vi "control_potencia_lentes.vi"() -> ()   [LabVIEW 2024]
uses:
  TG JD - running/TG Juan Diego/Documentos de Labview/160620 Optotune Lens Driver 4 Labview package/Hello Optotune Lens (30.06.2015)/Calibration.ctl
  <vilib>/Instr/_visa.llb/VISA Configure Serial Port (Instr).vi
  <vilib>/Utility/file.llb/Write Delimited Spreadsheet (string).vi
panel:
  out "potencia  DER 3":dbl[](graph)
  in  "Número Usuario 2":string
  out "potencia  DER 2":dbl[](graph)
  out "potencia  DER":dbl[](graph)
  out "x+1":i32
  in  "stop":bool
  in  "Tab Control":enum32{"Experimento", "Configuración"}(tab)
  out "Grabando DATOS":bool
  out "path":path
  in  "Genero":string(combo)
  in  "Potencia inicial lente derecho":dbl(slide) scale=-3.0..3.0
  in  "Potencia inicial lente izquierdo":dbl(slide) scale=-3.0..3.0
  in  "VISA resource name 2":string="COM10"
  in  "VISA resource name":string="COM11"
  in  "Carpeta":path=path "C:/Users/TGM1603/Documents/LabVIEW Data/Experimentos electrodos"
  in  "Edad":string
  in  "Número Usuario":string
  in  "Hipermetropía (?)":string(combo)
  in  "Miopía (?)":string(combo)
  out "error out 4":errorcluster
  out "error out 3":errorcluster
  out "DPT  DER":dbl
  in  "stop 4":bool
  in  "error in (no error) 3":errorcluster
  in  "error in (no error) 4":errorcluster
  out "DPT  IZQ":dbl
  in  "stop 3":bool
  out "VISA resource name out 2":string
  out "Command to Port":string
  out "Data":string
  out "OK":bool
  out "Calibration 2":T1 {"Max Current A" format="%#_g mA"; "Max Current B" format="%#_g mA"; "UCL A" format="%#_g mA"; "LCL A" format="%#_g mA"; "UCL B" format="%#_g mA"; "LCL B" format="%#_g mA"}
  out "VISA resource name out":string
  out "ID":u16
  in  "Calibration":T1={"Max Current A"=293.0, "Max Current B"=293.0, "UCL A"=300.0, "UCL B"=300.0, "LCL A"=0.0, "LCL B"=0.0} {"Max Current A" format="%#_g mA"; "Max Current B" format="%#_g mA"; "UCL A" format="%#_g mA"; "LCL A" format="%#_g mA"; "UCL B" format="%#_g mA"; "LCL B" format="%#_g mA"}
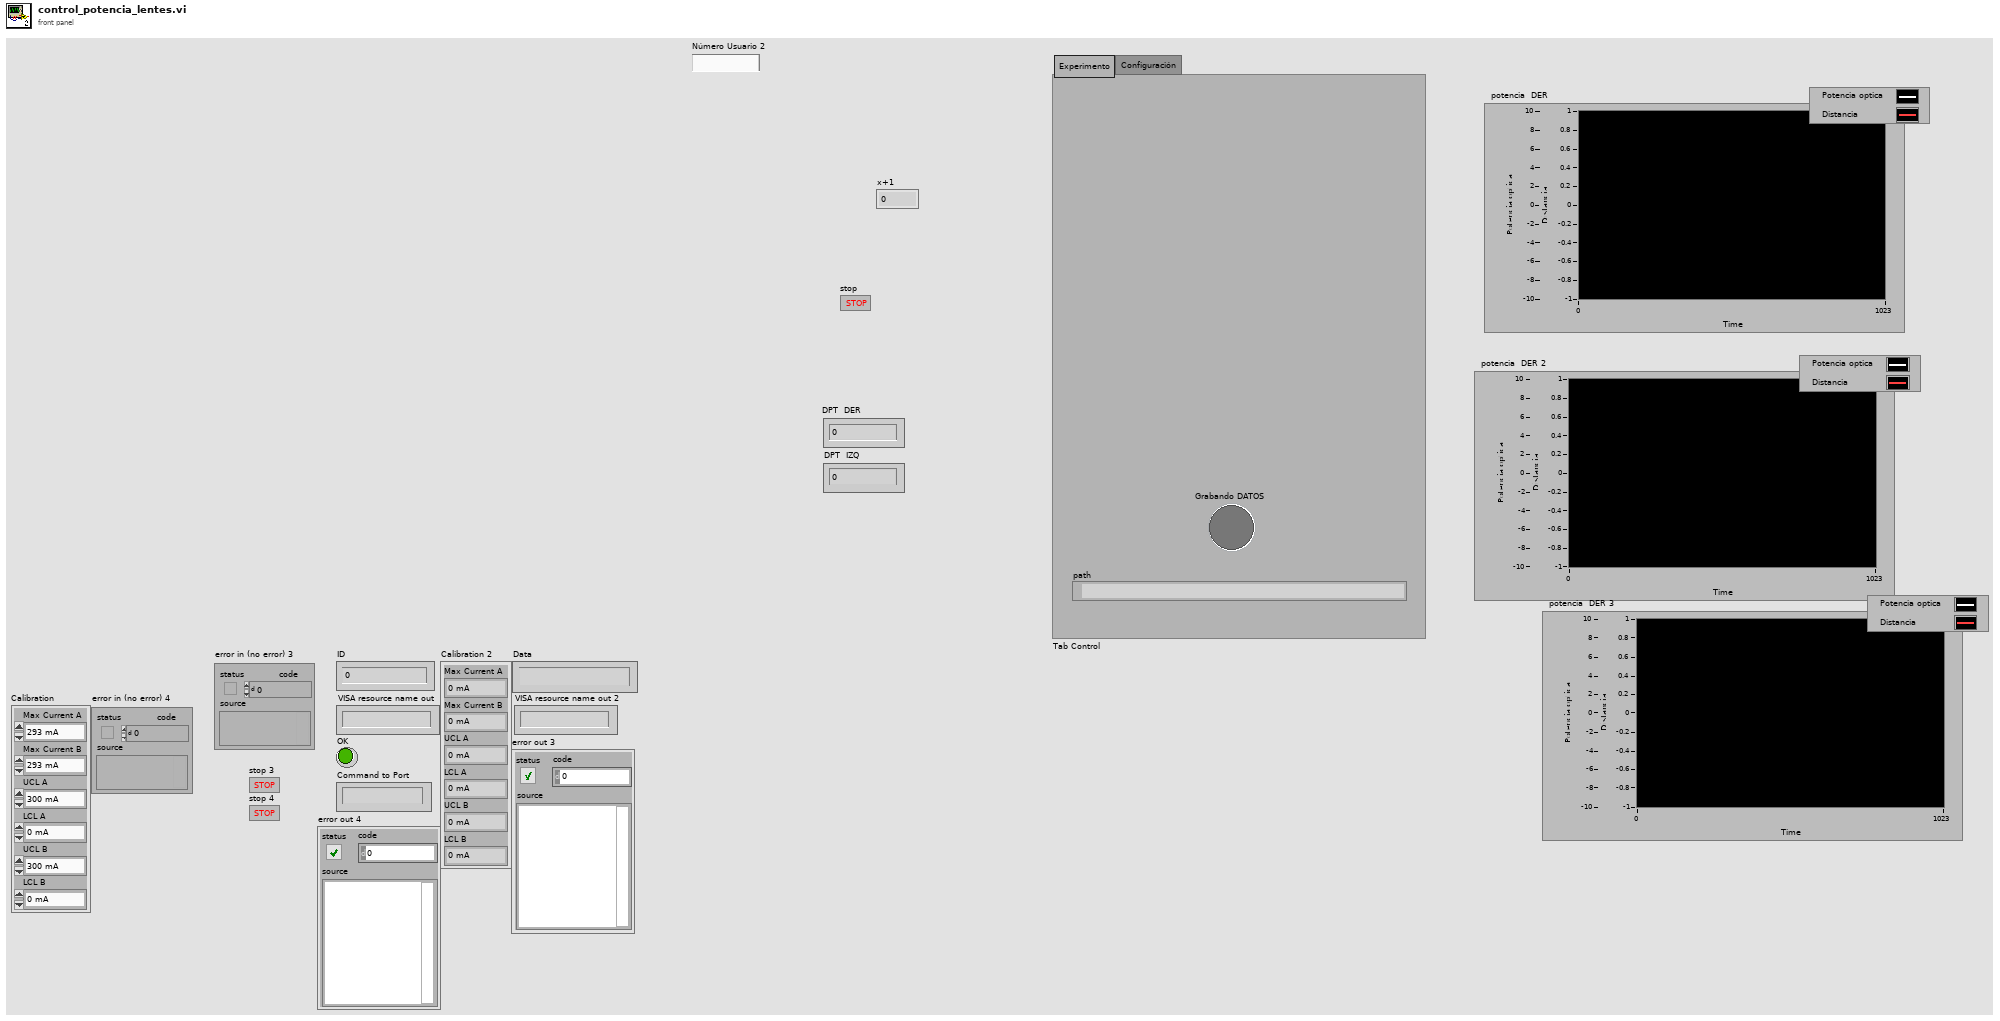
[diagram p1: front panel]
types:
  T1 = typedef "Calibration.ctl" = cluster{"Max Current A":dbl, "Max Current B":dbl, "UCL A":dbl, "UCL B":dbl, "LCL A":dbl, "LCL B":dbl}
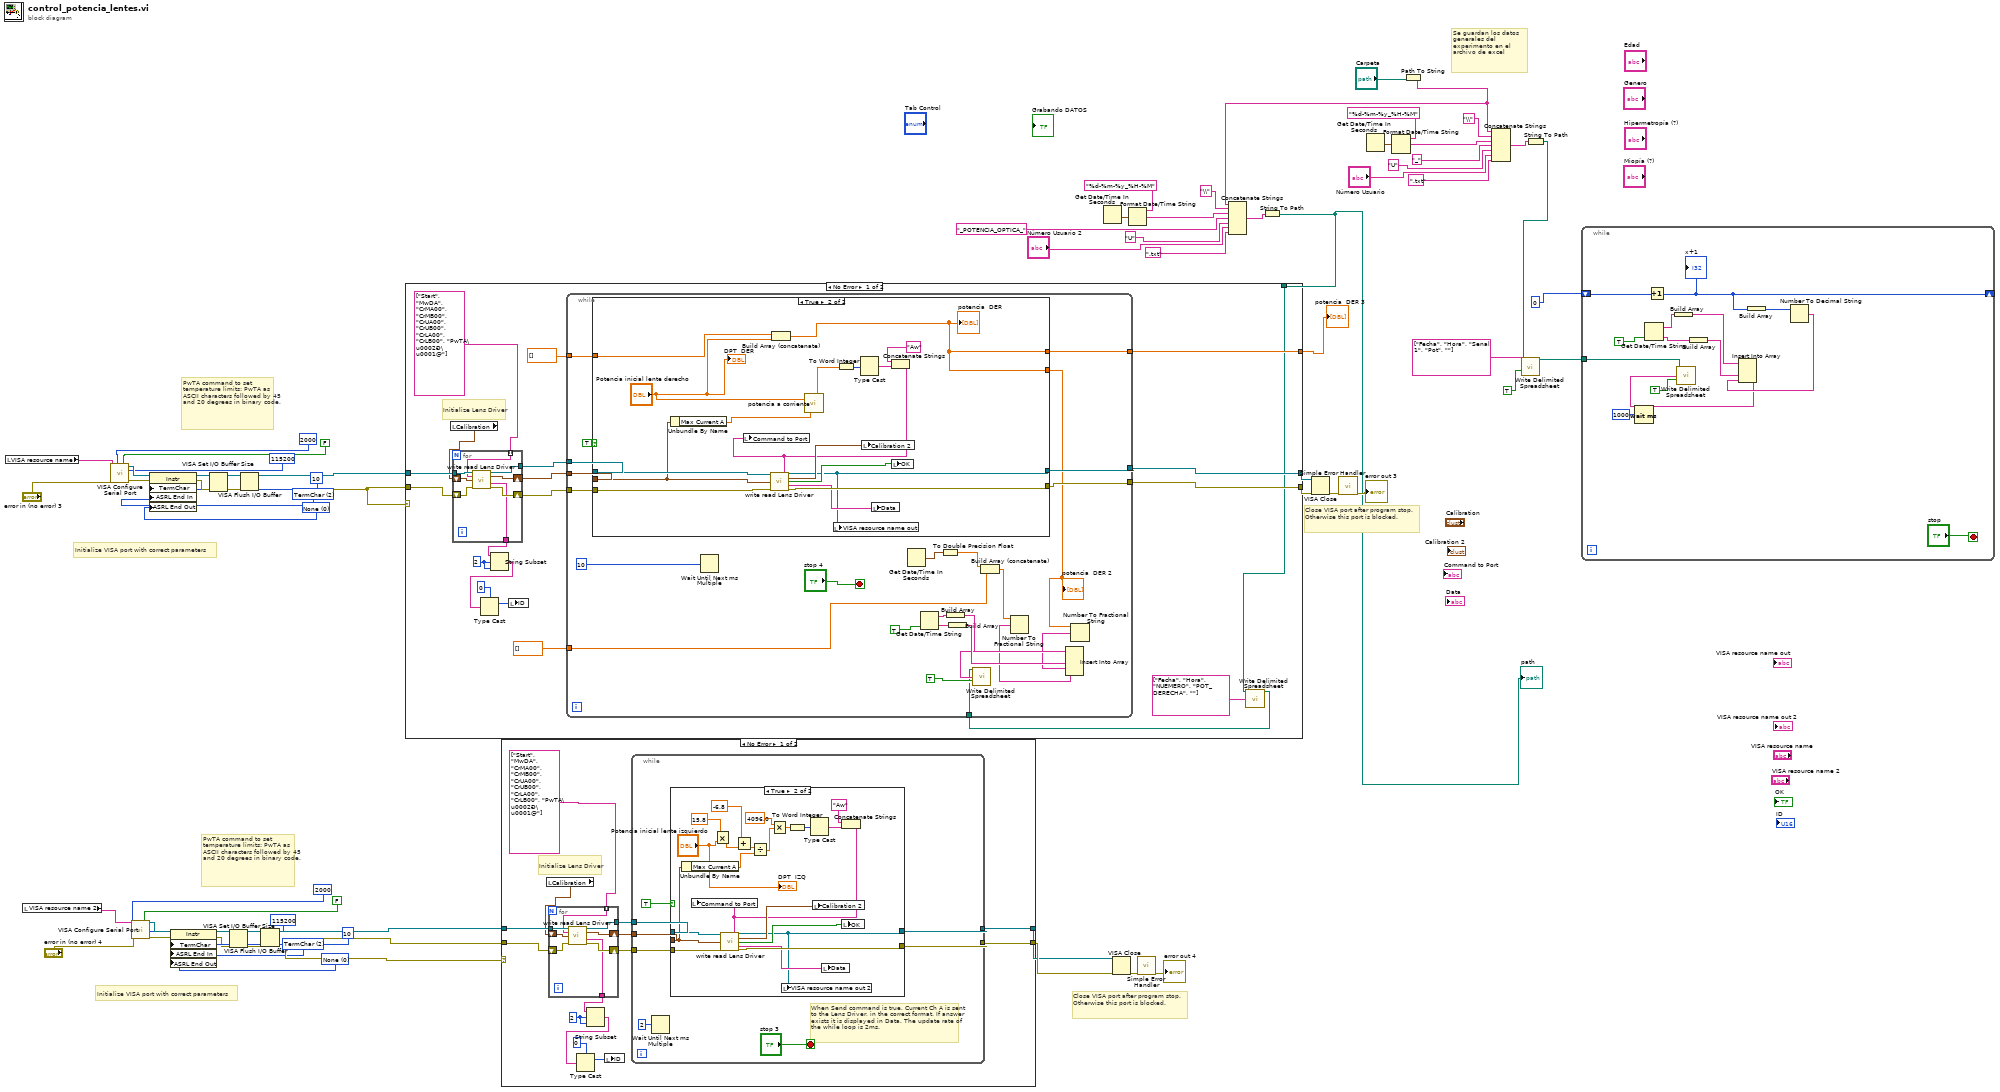
[diagram p0: block diagram]
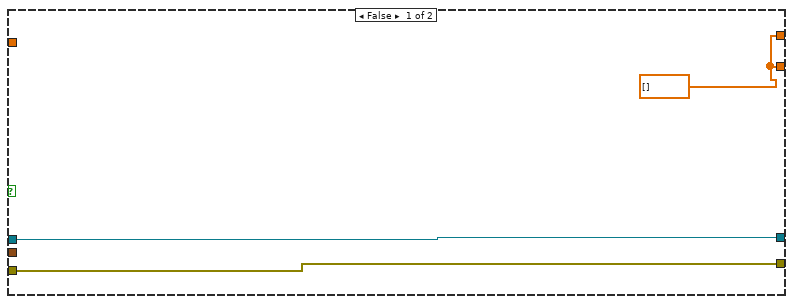
[diagram p2: hidden frame]
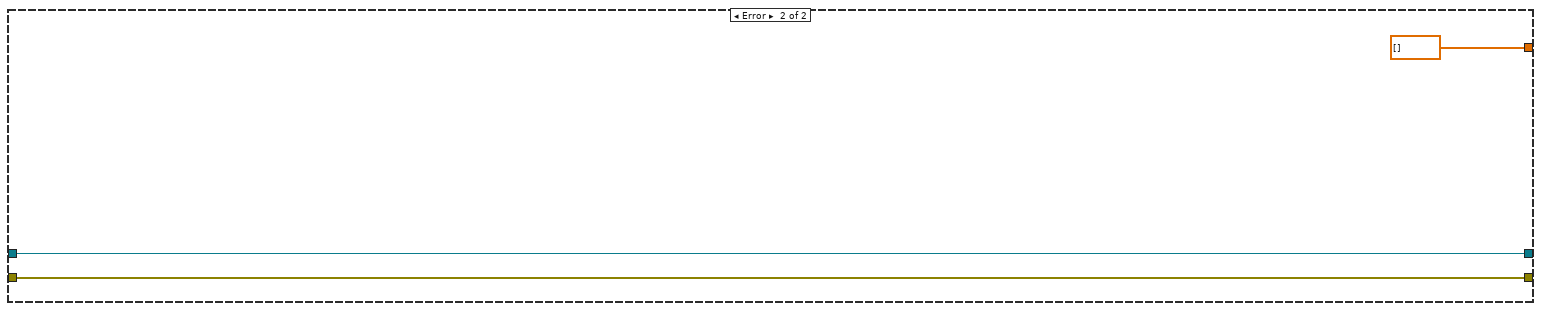
[diagram p3: hidden frame]
diagram:
  w48 = u16 0 items=["None", "Last Bit", "TermChar", "Break"] ("Serial Settings:End Mode for Writes")
  w47 = u16 2 items=["None", "Last Bit", "TermChar"] ("Serial Settings:End Mode for Reads")
  w61 = u16 0 items=["None", "Last Bit", "TermChar", "Break"] ("Serial Settings:End Mode for Writes")
  w60 = u16 2 items=["None", "Last Bit", "TermChar"] ("Serial Settings:End Mode for Reads")
  # "Se guardan los datos generales del experimento en el archivo de excel"
  # "Close VISA port after program stop. Otherwise this port is blocked."
  # "Close VISA port after program stop. Otherwise this port is blocked."
  # "PwTA command to set temperature limits: PwTA as ASCII characters followed by 45 and 20 degrees in binary code."
  # "Initialize VISA port with correct parameters"
  # "PwTA command to set temperature limits: PwTA as ASCII characters followed by 45 and 20 degrees in binary code."
  # "Initialize VISA port with correct parameters"
  n1 = local read "VISA resource name"() -> (w38:string)
  n2 = local read "VISA resource name 2"() -> (w52:string)
  n3 = call-poly "VISA Configure Serial Port"("VISA resource name"=w38, "timeout (10sec)"=u32 2000, "Enable Termination\nChar (T)"=FALSE ("Enable Termination\nChar (T)"), "baud rate (9600)"=u32 115200, "error in (no error)"="error in (no error) 3") -> ("VISA resource name out"=w43:refnum<visa-resource-name>, "error out"=w45:errorcluster)  [unwired: 9 in]
  n4 = call-poly "VISA Configure Serial Port"("VISA resource name"=w52, "timeout (10sec)"=u32 2000, "Enable Termination\nChar (T)"=FALSE ("Enable Termination\nChar (T)"), "baud rate (9600)"=u32 115200, "error in (no error)"="error in (no error) 4") -> ("VISA resource name out"=w56:refnum<visa-resource-name>, "error out"=w58:errorcluster)  [unwired: 9 in]
  n5 = property class="Instr"(reference=w43, error in=w45, "TermChar"=u8 10 ("Message Based Settings:Termination Character"), "ASRL End In"=w47, "ASRL End Out"=w48) -> (reference out=w44:refnum<visa-resource-name>, error out=w46:errorcluster)
  n6 = property class="Instr"(reference=w56, error in=w58, "TermChar"=u8 10 ("Message Based Settings:Termination Character"), "ASRL End In"=w60, "ASRL End Out"=w61) -> (reference out=w57:refnum<visa-resource-name>, error out=w59:errorcluster)
  n7 = VISA Set I/O Buffer Size(VISA resource name=w44, error in (no error)=w46) -> (VISA resource name out=w50:refnum<visa-resource-name>, error out=w51:errorcluster)  [unwired: 2 in]
  n8 = VISA Set I/O Buffer Size(VISA resource name=w57, error in (no error)=w59) -> (VISA resource name out=w63:refnum<visa-resource-name>, error out=w64:errorcluster)  [unwired: 2 in]
  n9 = VISA Flush I/O Buffer(VISA resource name=w50, error in (no error)=w51) -> (VISA resource name out=w37:refnum<visa-resource-name>, error out=w36:errorcluster)  [unwired: 1 in]
  n10 = VISA Flush I/O Buffer(VISA resource name=w63, error in (no error)=w64) -> (VISA resource name out=w66:refnum<visa-resource-name>, error out=w65:errorcluster)  [unwired: 1 in]
  n11 = case shown="No Error" w65 {
    tunnel: w65 -> [w81 w121]
    tunnel: w66 -> [w80 w122]
    tunnel: [w79 w121] -> w29
    tunnel: [w78 w122] -> w28
    frame No Error {
      w77 = 2 ("length (rest)")
      # "Initialize Lens Driver"
      n12 = local read "Calibration"() -> (w69:T1)
      n13 = for {
        tunnel: w80 -> [w119]
        tunnel: [w116] -> w72
        tunnel: string[] ["Start", "MwDA", "CrMA00", "CrMB00", "CrUA00", "CrUB00", "CrLA00", "CrLB00", "PwTA\u0002Ð\u0001@"] -> [w114] mode=indexing
        tunnel: [w113] -> w71
        shift-right: [w117] -> w73
        shift-left: w69 -> [w118]
        shift-right: [w115] -> w74
        shift-left: w81 -> [w120]
        n14 = call "write read Lens Driver.vi"("VISA resource name"=w119, "command"=w114, "Calibration"=w118, "error in (no error)"=w120) -> ("VISA resource name out"=w116:refnum<visa-resource-name>, "Calibration 2"=w117:T1, "Data"=w113:string, "error out"=w115:errorcluster)  [unwired: 4 in, 4 out]
      }
      n15 = String Subset(string=w71, offset (0)=w77, length (rest)=w77) -> (substring=w75:string)
      n16 = Type Cast(type=u16 0 ("length (rest)"), x=w75) -> (*(type *) &x=w70:u16)
      n17 = local write "ID"(w70) -> ()
      n18 = while {
        tunnel: [w83] -> w79
        tunnel: [w84] -> w78
        tunnel: w74 -> [w89]
        tunnel: w73 -> [w88]
        tunnel: w72 -> [w87]
        stop <- "stop 3" stop-if-true
        # "When Send command is true, Current Ch A is sent to the Lens Driver, in the correct format. If answer exists it is displayed in Data. The update rate of the while loop is 2ms."
        n19 = Wait Until Next ms Multiple(millisecond multiple=u32 2) -> ()  [unwired: 1 out]
        n20 = case shown="True" TRUE ("Send command") {
          tunnel: [w91 w112] -> w83
          tunnel: w89 -> [w91 w111]
          tunnel: w88 -> [_ w99]
          tunnel: w87 -> [w90 w110]
          tunnel: [w90 w100] -> w84
          frame False {
          }
          frame True {
            n21 = Unbundle By Name(w99) -> ("Max Current A"=w98:dbl)
            n22 = Multiply(x=15.8, y="Potencia inicial lente izquierdo") -> (x*y=w96:dbl)
            n23 = Add(x=-6.8, y=w96) -> (x+y=w94:dbl)
            n24 = Divide(x=w94, y=w98) -> (x/y=w97:dbl)
            n25 = Multiply(x=4096.0, y=w97) -> (x*y=w108:dbl)
            n26 = To Word Integer(number=w108) -> (16bit integer=w107:i16)
            n27 = Type Cast(x=w107) -> (*(type *) &x=w106:string)  [unwired: 1 in]
            n28 = Concatenate Strings("Aw", w106) -> (w102:string)
            n29 = local write "Command to Port"(w102) -> ()
            n30 = call "write read Lens Driver.vi"("VISA resource name"=w110, "command"=w102, "Calibration"=w99, "error in (no error)"=w111) -> ("VISA resource name out"=w100:refnum<visa-resource-name>, "Calibration 2"=w104:T1, "OK"=w103:bool, "Data"=w101:string, "error out"=w112:errorcluster)  [unwired: 4 in, 3 out]
            n31 = local write "VISA resource name out 2"(w100) -> ()
            n32 = local write "Calibration 2"(w104) -> ()
            n33 = local write "Data"(w101) -> ()
            n34 = local write "OK"(w103) -> ()
            "DPT  IZQ" <- "Potencia inicial lente izquierdo"
          }
        }
      }
    }
    frame Error {
    }
  }
  n35 = Get Date/Time In Seconds() -> (seconds since 1Jan1904=w13:timestamp)
  n36 = VISA Close(VISA resource name=w28, error in (no error)=w29) -> (error out=w31:errorcluster)
  n37 = Format Date/Time String(time format string (%c)="%d-%m-%y_%H-%M", seconds (now)=w13) -> (date/time string=w9:string)  [unwired: 1 in]
  n38 = call <vilib>:"Simple Error Handler.vi"("error in (no error)"=w31) -> ("error out"=→"error out 4":errorcluster)  [unwired: 4 in, 4 out]
  n39 = Get Date/Time In Seconds() -> (seconds since 1Jan1904=w27:timestamp)
  n40 = Format Date/Time String(time format string (%c)="%d-%m-%y_%H-%M", seconds (now)=w27) -> (date/time string=w22:string)  [unwired: 1 in]
  n41 = Path To String(path="Carpeta") -> (string=w4:string)
  n42 = Concatenate Strings(w4, "\\" ("string"), w9, "_POTENCIA_OPTICA_" ("string"), "U" ("string"), "Número Usuario 2", ".txt" ("string")) -> (w10:string)
  n43 = String To Path(string=w10) -> (path=w1:path)
  "path" <- w1
  n44 = case shown="No Error" w36 {
    tunnel: w36 -> [w142 w197]
    tunnel: w37 -> [w141 w198]
    tunnel: [w140 w197] -> w32
    tunnel: [w139 w198] -> w33
    tunnel: [w127 dbl[] []] -> w2
    tunnel: w1 -> [w126 _]
    frame No Error {
      w138 = 2 ("length (rest)")
      # "Initialize Lens Driver"
      n45 = local read "Calibration"() -> (w130:T1)
      n46 = for {
        tunnel: w141 -> [w194]
        tunnel: [w191] -> w133
        tunnel: string[] ["Start", "MwDA", "CrMA00", "CrMB00", "CrUA00", "CrUB00", "CrLA00", "CrLB00", "PwTA\u0002Ð\u0001@"] -> [w189] mode=indexing
        tunnel: [w188] -> w132
        shift-right: [w192] -> w134
        shift-left: w130 -> [w193]
        shift-right: [w190] -> w135
        shift-left: w142 -> [w195]
        n47 = call "write read Lens Driver.vi"("VISA resource name"=w194, "command"=w189, "Calibration"=w193, "error in (no error)"=w195) -> ("VISA resource name out"=w191:refnum<visa-resource-name>, "Calibration 2"=w192:T1, "Data"=w188:string, "error out"=w190:errorcluster)  [unwired: 4 in, 4 out]
      }
      n48 = String Subset(string=w132, offset (0)=w138, length (rest)=w138) -> (substring=w136:string)
      n49 = Type Cast(type=u16 0 ("length (rest)"), x=w136) -> (*(type *) &x=w131:u16)
      n50 = local write "ID"(w131) -> ()
      n51 = call-poly <vilib>:"Write Delimited Spreadsheet.vi"("file path (dialog if empty)"=w126, "1D data"=string[] ["Fecha", "Hora", "NUEMERO", "POT_DERECHA", ""]) -> ("new file path (Not A Path if cancelled)"=w124:path)  [unwired: 12 in, 1 out]
      n52 = while {
        tunnel: [w161] -> w140
        tunnel: [w162] -> w139
        tunnel: w135 -> [w167]
        tunnel: w134 -> [w166]
        tunnel: w133 -> [w165]
        tunnel: dbl[] [] -> [w159]
        tunnel: [w158] -> w127
        tunnel: w124 -> [w150]
        tunnel: dbl[] [] -> [w143]
        stop <- "stop 4" stop-if-true
        n53 = case shown="True" TRUE ("Send command") {
          tunnel: [w170 w187] -> w161
          tunnel: w167 -> [w170 w186]
          tunnel: w166 -> [_ w177]
          tunnel: w165 -> [w169 w185]
          tunnel: [w169 w178] -> w162
          tunnel: w159 -> [_ w172]
          tunnel: [w168 w171] -> w148
          tunnel: [w168 w171] -> w158
          frame False {
            w168 = dbl[] []
          }
          frame True {
            n54 = Unbundle By Name(w177) -> ("Max Current A"=w176:dbl)
            n55 = Build Array (concatenate)(w172, "Potencia inicial lente derecho") -> (w171:dbl[])
            "potencia  DER" <- w171
            n56 = call "potencia a corriente.vi"("Max current A"=w176, "Potencia"="Potencia inicial lente derecho") -> ("Corriente"=w175:dbl)
            n57 = To Word Integer(number=w175) -> (16bit integer=w184:i16)
            n58 = Type Cast(x=w184) -> (*(type *) &x=w183:string)  [unwired: 1 in]
            n59 = Concatenate Strings("Aw", w183) -> (w180:string)
            n60 = local write "Command to Port"(w180) -> ()
            n61 = call "write read Lens Driver.vi"("VISA resource name"=w185, "command"=w180, "Calibration"=w177, "error in (no error)"=w186) -> ("VISA resource name out"=w178:refnum<visa-resource-name>, "Calibration 2"=w182:T1, "OK"=w181:bool, "Data"=w179:string, "error out"=w187:errorcluster)  [unwired: 4 in, 3 out]
            n62 = local write "VISA resource name out"(w178) -> ()
            n63 = local write "Calibration 2"(w182) -> ()
            n64 = local write "Data"(w179) -> ()
            n65 = local write "OK"(w181) -> ()
            "DPT  DER" <- "Potencia inicial lente derecho"
          }
        }
        "potencia  DER 2" <- w148
        n66 = Wait Until Next ms Multiple(millisecond multiple=u32 10) -> ()  [unwired: 1 out]
        n67 = Get Date/Time In Seconds() -> (seconds since 1Jan1904=w145:timestamp)
        n68 = Get Date/Time String(want seconds? (F)=TRUE) -> (date string=w157:string, time string=w156:string)  [unwired: 2 in]
        n69 = To Double Precision Float(number=w145) -> (double precision float=w144:dbl)
        n70 = Build Array(w157) -> (w155:string[])
        n71 = Build Array(w156) -> (w154:string[])
        n72 = Build Array (concatenate)(w144, w143) -> (w147:dbl[])
        n73 = Number To Fractional String(number=w147) -> (F-format string=w146:string[])  [unwired: 3 in]
        n74 = Number To Fractional String(number=w148) -> (F-format string=w149:string[])  [unwired: 3 in]
        n75 = Insert Into Array(array=w155, new element #1=w154, new element #2=w149, new element #3=w146) -> (w153:string[])  [unwired: 1 in]
        n76 = call-poly <vilib>:"Write Delimited Spreadsheet.vi"("file path (dialog if empty)"=w150, "1D data"=w153, "append to file? (new file:F)"=TRUE) -> ()  [unwired: 11 in, 2 out]
      }
    }
    frame Error {
    }
  }
  "potencia  DER 3" <- w2
  n77 = VISA Close(VISA resource name=w33, error in (no error)=w32) -> (error out=w35:errorcluster)
  n78 = call <vilib>:"Simple Error Handler.vi"("error in (no error)"=w35) -> ("error out"=→"error out 3":errorcluster)  [unwired: 4 in, 4 out]
  n79 = Concatenate Strings(w4, "\\" ("string"), w22, "_" ("string"), "U" ("string"), "Número Usuario", ".txt" ("string")) -> (w23:string)
  n80 = String To Path(string=w23) -> (path=w3:path)
  n81 = call-poly <vilib>:"Write Delimited Spreadsheet.vi"("file path (dialog if empty)"=w3, "1D data"=string[] ["Fecha", "Hora", "Senal 1", "Pot", ""], "append to file? (new file:F)"=TRUE) -> ("new file path (Not A Path if cancelled)"=w15:path)  [unwired: 11 in, 1 out]
  n82 = while {
    shift-right: [w207] -> _
    shift-left: 0 -> [w212]
    tunnel: w15 -> [w202]
    stop <- "stop" stop-if-true
    n83 = Wait (ms)(milliseconds to wait=u32 1000) -> ()  [unwired: 1 out]
    n84 = Get Date/Time String(want seconds? (F)=TRUE) -> (date string=w209:string, time string=w208:string)  [unwired: 2 in]
    n85 = Increment(x=w212) -> (x+1=w207:i32)
    "x+1" <- w207
    n86 = Build Array(w209) -> (w206:string[])
    n87 = Build Array(w208) -> (w205:string[])
    n88 = Build Array(w207) -> (w204:i32[])
    n89 = Number To Decimal String(number=w204) -> (decimal integer string=w203:string[])  [unwired: 1 in]
    n90 = Insert Into Array(array=w206, new element #1=w205, new element #2=w203) -> (w201:string[])  [unwired: 1 in]
    n91 = call-poly <vilib>:"Write Delimited Spreadsheet.vi"("file path (dialog if empty)"=w202, "1D data"=w201, "append to file? (new file:F)"=TRUE) -> ()  [unwired: 11 in, 2 out]
  }
